vi "CRYGet Window Temp Reference.vi"(8 "sWindowName":string, 9 "sVIFullName":path, 10 "pVIRef_In":refnum<vi>, 11 "sAction":string) -> (0 "bResult":bool=TRUE, 1 "nWinType":i32, 2 "sTitleName Out":string, 3 "pVIRef_Out":refnum<vi>, 4 "sIcon_Out":string)   [LabVIEW 2013]
uses:
  <vilib>/Utility/miscctls.llb/LVPointTypeDef.ctl
  CRYWindow/SubVI/CRYMain Sub Window Global.vi
  Program/CRYRef nums global.vi
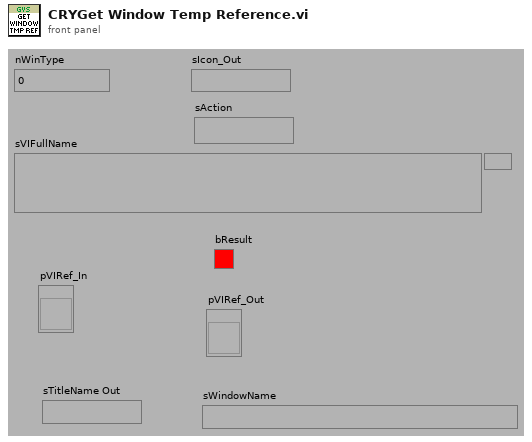
[diagram p1: front panel]
types:
  T1 = enum32{"Invalid", "Default", "Floating", "Floating/Auto-Hide", "Modal"}
  T2 = enum32{"Invalid", "Standard", "Closed", "Hidden", "Minimized", "Maximized"}
  T3 = typedef "LVPointTypeDef.ctl" = cluster{"Horizontal":i16, "Vertical":i16}
  T4 = cluster{"CLOSE_HIDE":i32, "CLOSE_CLOSE":i32, "DOCK_ENABLE":i32, "DOCK_DISABLE":i32, "FOCUS_SHOW":i32, "FOCUS_HIDE":i32}
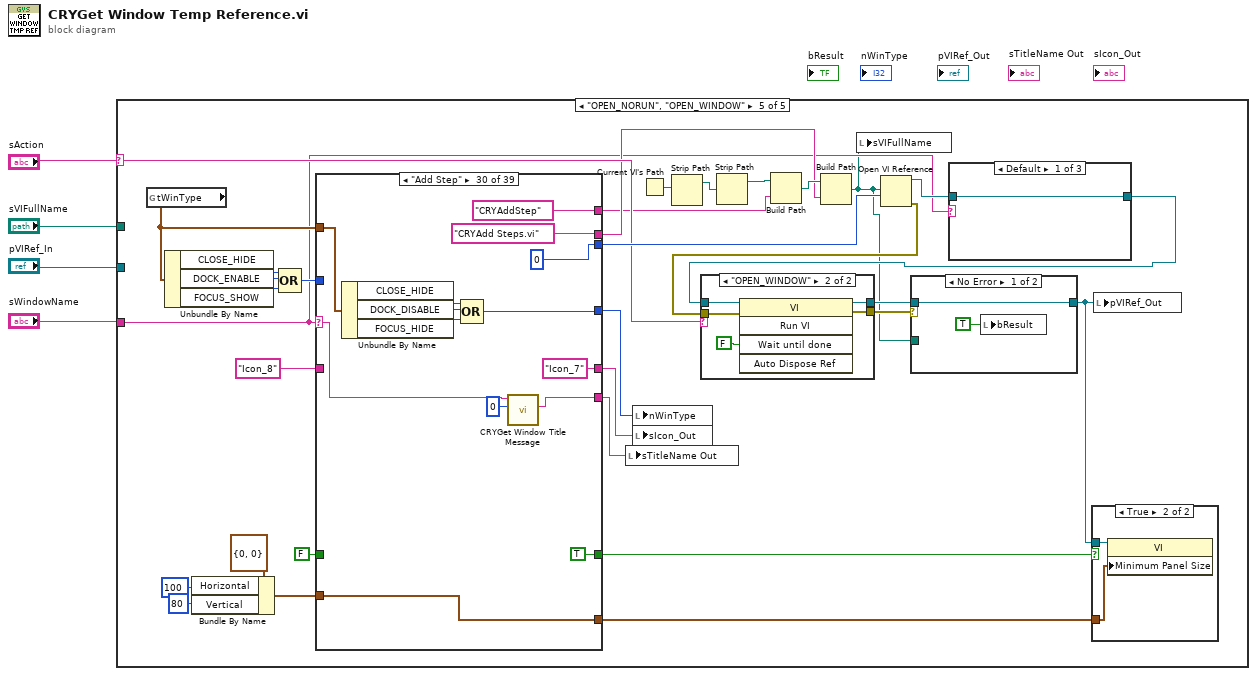
[diagram p0: block diagram]
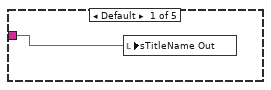
[diagram p2: hidden frame]
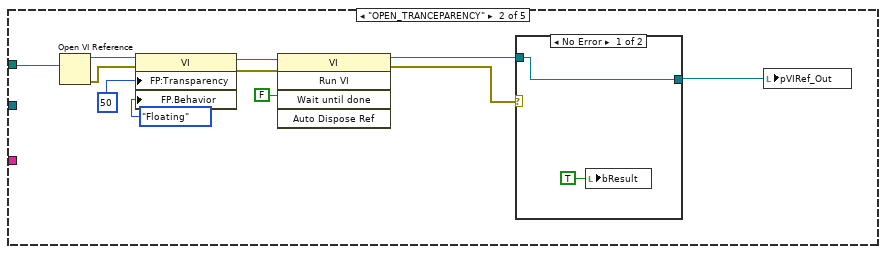
[diagram p3: hidden frame]
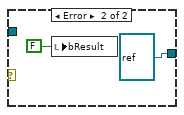
[diagram p4: hidden frame]
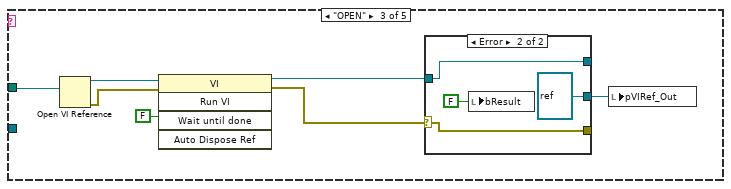
[diagram p5: hidden frame]
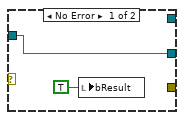
[diagram p6: hidden frame]
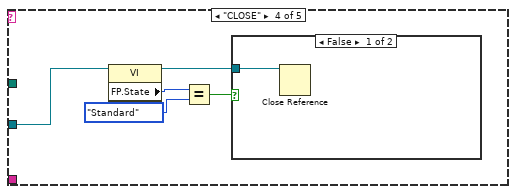
[diagram p7: hidden frame]
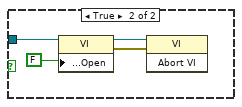
[diagram p8: hidden frame]
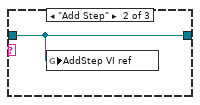
[diagram p9: hidden frame]
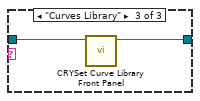
[diagram p10: hidden frame]
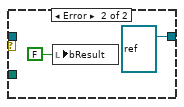
[diagram p13: hidden frame]
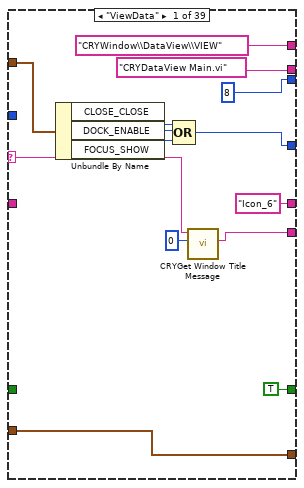
[diagram p14: hidden frame]
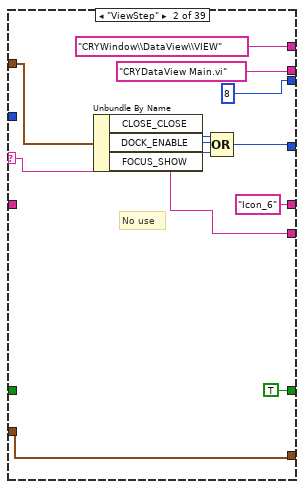
[diagram p15: hidden frame]
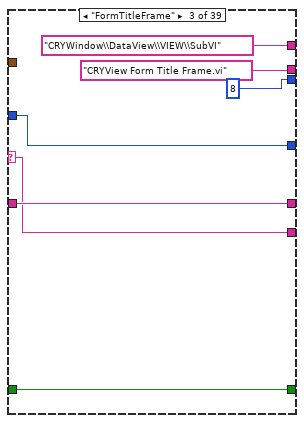
[diagram p16: hidden frame]
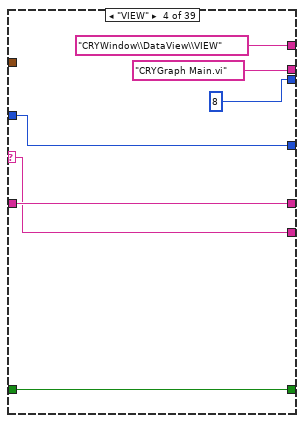
[diagram p17: hidden frame]
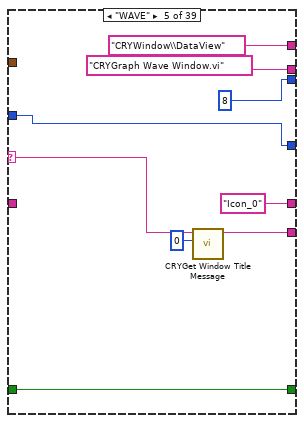
[diagram p18: hidden frame]
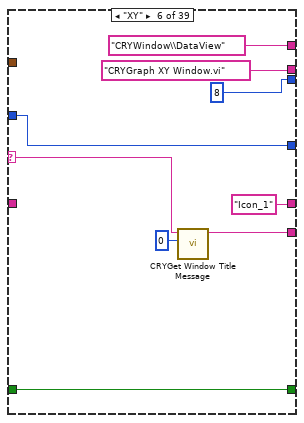
[diagram p19: hidden frame]
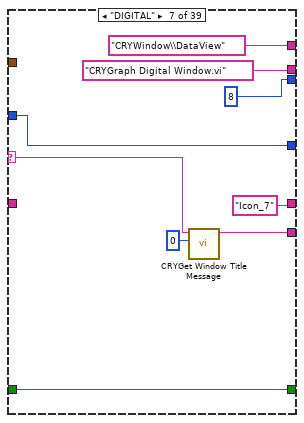
[diagram p20: hidden frame]
diagram:
  n1 = case shown="\"OPEN_NORUN\", \"OPEN_WINDOW\"" "sAction" {
    selector: "sAction" -> [_ _ _ _ w63]
    tunnel: "sVIFullName" -> [_ w7 w24 _ _]
    tunnel: "pVIRef_In" -> [_ _ _ w36 _]
    tunnel: "sWindowName" -> [w5 _ _ _ w48]
    frame Default {
      n2 = local write "sTitleName Out"(w5) -> ()
    }
    frame "OPEN_TRANCEPARENCY" {
      n3 = Open VI Reference(vi path=w7) -> (vi reference=w12:refnum<vi>, error out=w13:errorcluster)  [unwired: 1 in, 4 out]
      n4 = property class="VI"(reference=w12, error in=w13, "FP:Transparency"=u8 50 ("Front Panel Window:Transparency"), "FP.Behavior"=T1."Floating" ("Front Panel Window:Behavior")) -> (reference out=w15:refnum<vi>, error out=w16:errorcluster)
      n5 = invoke class="VI" method="Run VI"(reference=w15, error in=w16, "Wait until done"=FALSE ("Wait Until Done")) -> (reference out=w8:refnum<vi>, error out=w9:errorcluster)  [unwired: 2 in, 3 out]
      n6 = case shown="No Error" w9 {
        tunnel: w8 -> [w17 _]
        tunnel: [w17 refnum<vi> refnum ("VIRef")] -> w6
        frame No Error {
          n7 = local write "bResult"(TRUE ("bResult")) -> ()
        }
        frame Error {
          n8 = local write "bResult"(FALSE ("bResult")) -> ()
        }
      }
      n9 = local write "pVIRef_Out"(w6) -> ()
    }
    frame "OPEN" {
      n10 = Open VI Reference(vi path=w24) -> (vi reference=w23:refnum<vi>, error out=w22:errorcluster)  [unwired: 1 in, 4 out]
      n11 = invoke class="VI" method="Run VI"(reference=w23, error in=w22, "Wait until done"=FALSE ("Wait Until Done")) -> (reference out=w25:refnum<vi>, error out=w26:errorcluster)  [unwired: 2 in, 3 out]
      n12 = case shown="Error" w26 {
        selector: w26 -> [_ w30]
        tunnel: w25 -> [w28 w31]
        tunnel: [w28 refnum<vi> refnum ("VIRef_Out")] -> w21
        tunnel: [_ w31] -> _
        tunnel: [_ w30] -> _
        frame No Error {
          n13 = local write "bResult"(TRUE ("bResult")) -> ()
        }
        frame Error {
          n14 = local write "bResult"(FALSE ("bResult")) -> ()
        }
      }
      n15 = local write "pVIRef_Out"(w21) -> ()
    }
    frame "CLOSE" {
      n16 = property class="VI"(reference=w36) -> (reference out=w34:refnum<vi>, "FP.State"=w38:T2)  [unwired: 1 in, 1 out]
      n17 = Equal?(x=w38, y=T2."Standard" ("Front Panel Window:State")) -> (x = y?=w35:bool)
      n18 = case shown="False" w35 {
        tunnel: w34 -> [w39 w42]
        frame False {
          n19 = Close Reference(reference=w39) -> ()  [unwired: 1 in, 1 out]
        }
        frame True {
          n20 = property class="VI"(reference=w42, "Front Panel.Open"=FALSE ("Front Panel Window:Open")) -> (reference out=w41:refnum<vi>, error out=w40:errorcluster)  [unwired: 1 in]
          n21 = invoke class="VI" method="Abort VI"(reference=w41, error in=w40) -> ()  [unwired: 1 in, 3 out]
        }
      }
    }
    frame "OPEN_NORUN", "OPEN_WINDOW" {
      n22 = global read "CRYMain Sub Window Global.vi" "tWinType"() -> (w61:T4)
      n23 = Unbundle By Name(w61) -> ("CLOSE_HIDE"=w68:i32, "DOCK_ENABLE"=w69:i32, "FOCUS_SHOW"=w70:i32)
      n24 = Bundle By Name(cluster=T3 {"Horizontal"=0, "Vertical"=0} ("Front Panel Window:Minimum Size"), "Horizontal"=i16 100, "Vertical"=i16 80) -> (w52:T3)
      n25 = Compound Arithmetic op=OR(w68, w69, w70) -> (w67:i32)
      n26 = case shown="\"Add Step\"" w48 {
        selector: w48 -> [w97 w109 w120 w128 w135 w144 w153 w162 w171 w180 w189 w198 w207 w216 w226 w234 w246 w259 w269 w279 w286 w293 w300 w309 w317 w328 w339 w350 w361 w370 w382 w391 w403 w410 w417 w424 w431 w438 w445]
        tunnel: ["CRYWindow\\DataView\\VIEW" ("name") "CRYWindow\\DataView\\VIEW" ("name") "CRYWindow\\DataView\\VIEW\\SubVI" ("name") "CRYWindow\\DataView\\VIEW" ("name") "CRYWindow\\DataView" ("name") "CRYWindow\\DataView" ("name") "CRYWindow\\DataView" ("name") "CRYWindow\\DataView" ("name") "CRYWindow\\DataView" ("name") "CRYWindow\\DataView" ("name") "CRYWindow\\DataView" ("name") "CRYWindow\\DataView" ("name") "CRYWindow\\DataView" ("name") "CRYWindow\\DataView" ("name") "CRYStepSetup" ("name") "CRYStepSetup" ("name") "CRYDocument" ("name") "CRYDocument" ("name") "CRYCurveLibrary" ("name") "CRYCurveLibrary\\SubVI" ("name") "CRYCurveLibrary\\SubVI" ("name") "CRYCurveLibrary\\SubVI" ("name") "CRYCurveLibrary\\SubVI" ("name") "CRYProject" ("name") "CRYSystem\\Misc" ("name") "CRYSystem\\Misc" ("name") "CRYSystem\\Misc" ("name") "CRYSystem\\Misc" ("name") "CRYWindow\\SubVI" ("name") "CRYAddStep" ("name") "CRYOne\\" ("name") "CRYOne" ("name") "CRYWindow\\SubVI" ("name") "CRYWindow\\SubVI" ("name") "CRYWindow\\SubVI" ("name") "CRYWindow\\SubVI" ("name") "CRYWindow\\SubVI" ("name") "CRYSystem\\Misc" ("name") "CRYWindow\\SubVI" ("name")] -> w51
        tunnel: ["CRYDataView Main.vi" ("name") "CRYDataView Main.vi" ("name") "CRYView Form Title Frame.vi" ("name") "CRYGraph Main.vi" ("name") "CRYGraph Wave Window.vi" ("name") "CRYGraph XY Window.vi" ("name") "CRYGraph Digital Window.vi" ("name") "CRYGraph Octave Window.vi" ("name") "CRYGraph Polar Window.vi" ("name") "CRYGraph Text Window.vi" ("name") "CRYGraph Table Window.vi" ("name") "CRYGraph Picture Window.vi" ("name") "CRYGraph Result Window.vi" ("name") "CRYGraph Intensity Window.vi" ("name") "CRYStepSetup.vi" ("name") "CRYStep Setup Default Window.vi" ("name") "CRYReport Main.vi" ("name") "SubVI\\CRYReport Frame.vi" ("name") "CRYCurve Library.vi" ("name") "CRYProbe Curve.vi" ("name") "CRYProbe Value.vi" ("name") "CRYProbe Result.vi" ("name") "CRYProbe Waveform.vi" ("name") "CRYProject Editor.vi" ("name") "CRYSignal Generator.vi" ("name") "CRYMultimeter.vi" ("name") "CRYScope-FFT.vi" ("name") "CRYRTA.vi" ("name") "CRYAPI TAB MAIN.vi" ("name") "CRYAdd Steps.vi" ("name") "CRYOne Quick Lunch Menu.vi" ("name") "CRYSequence Generator.vi" ("name") "CRYAPI Splitter Vertical.vi" ("name") "CRYAPI Splitter Horizontal.vi" ("name") "CRYAPI Temp Empty.vi" ("name") "CRYAPI Temp Frame.vi" ("name") "CRYAPI MSG PRO.vi" ("name") "CRYOperator Message.vi" ("name") "CRYAPI Temp Default.vi" ("name")] -> w60
        tunnel: [w99 w110 w123 w131 w140 w149 w158 w166 w175 w184 w193 w202 w211 w220 w228 w238 w248 w263 w272 w282 w289 w295 w303 w313 w318 w329 w340 w351 w364 w374 w385 w395 w406 0 w420 w427 w434 w441 w448] -> w71
        tunnel: w67 -> [_ _ w123 w131 w140 w149 w158 w166 w175 w184 w193 w202 w211 w220 w228 w238 _ w263 w272 w282 w289 w295 w303 w313 _ _ _ _ w364 _ w385 _ w406 _ w420 w427 w434 w441 w448]
        tunnel: "Icon_8" ("sIcon_Out") -> [_ _ w122 w130 _ _ _ _ _ _ _ _ _ _ _ w237 _ _ _ w281 w287 w294 w301 _ _ _ _ _ w363 _ w383 _ w405 w412 w419 w426 w433 w440 w447]
        tunnel: ["Icon_6" ("sIcon_Out") "Icon_6" ("sIcon_Out") w122 w130 "Icon_0" ("sIcon_Out") "Icon_1" ("sIcon_Out") "Icon_7" ("sIcon_Out") "Icon_5" ("sIcon_Out") "Icon_2" ("sIcon_Out") "Icon_6" ("sIcon_Out") "Icon_3" ("sIcon_Out") "Icon_8" ("sIcon_Out") "Icon_4" ("sIcon_Out") "Icon_9" ("sIcon_Out") "Icon_3" ("sIcon_Out") w237 "Icon_4" ("sIcon_Out") "Icon_6" ("sIcon_Out") w264 w281 w287 w294 w301 "Icon_1" ("sIcon_Out") "Icon_8" ("sIcon_Out") "Icon_8" ("sIcon_Out") "Icon_8" ("sIcon_Out") "Icon_8" ("sIcon_Out") w363 "Icon_7" ("sIcon_Out") w383 "Icon_7" ("sIcon_Out") w405 w412 w419 w426 w433 w440 w447] -> w65
        tunnel: [8 ("options") 8 ("options") 8 ("options") 8 ("options") 8 ("options") 8 ("options") 8 ("options") 8 ("options") 8 ("options") 8 ("options") 8 ("options") 8 ("options") 8 ("options") 8 ("options") 8 ("options") 8 ("options") 8 ("options") 8 ("options") 0 ("options") 8 ("options") 8 ("options") 8 ("options") 8 ("options") 0 ("options") 8 ("options") 8 ("options") 8 ("options") 8 ("options") 8 ("options") 0 ("options") 0 ("options") 0 ("options") 8 ("options") 8 ("options") 8 ("options") 8 ("options") 8 ("options") 0 ("options") 8 ("options")] -> w64
        tunnel: w61 -> [w100 w111 _ _ _ _ _ _ _ _ _ _ _ _ _ _ w249 _ _ _ _ _ _ _ w319 w330 w341 w352 _ w375 _ w396 _ _ _ _ _ _ _]
        tunnel: [w96 w109 w120 w128 w133 w142 w151 w160 w169 w178 w187 w196 w205 w214 w225 w234 w245 w259 w268 w279 w286 w293 w300 w308 w317 w328 w339 w350 w361 w369 w382 w390 w403 w410 w417 w424 w431 w438 w445] -> w62
        tunnel: FALSE -> [_ _ w119 w127 w134 w143 w152 w161 w170 w179 w188 w197 w206 w215 _ w233 _ w257 _ w278 w285 w292 w299 _ w316 w327 w338 w349 w360 _ w381 _ w402 w409 w416 w423 w430 w437 w444]
        tunnel: [TRUE TRUE w119 w127 w134 w143 w152 w161 w170 w179 w188 w197 w206 w215 TRUE w233 TRUE w257 TRUE w278 w285 w292 w299 TRUE w316 w327 w338 w349 w360 TRUE w381 TRUE w402 w409 w416 w423 w430 w437 w444] -> w57
        tunnel: [w94 w107 _ _ _ _ _ _ _ _ _ _ _ _ w223 _ w241 _ w266 _ _ _ _ w306 _ _ _ _ _ w367 _ w388 _ _ _ _ _ _ _] -> w56
        tunnel: w52 -> [w94 w107 _ _ _ _ _ _ _ _ _ _ _ _ w223 _ _ _ w266 _ _ _ _ w306 _ _ _ _ _ w367 _ w388 _ _ _ _ _ _ _]
        frame "ViewData" {
          n27 = Unbundle By Name(w100) -> ("CLOSE_CLOSE"=w103:i32, "DOCK_ENABLE"=w102:i32, "FOCUS_SHOW"=w101:i32)
          n28 = Compound Arithmetic op=OR(w103, w102, w101) -> (w99:i32)
          n29 = call "CRYGet Window Title Message.vi"("No"=0 ("Error No"), "Kind"=w97) -> ("Unicode String"=w96:string)  [unwired: 4 in, 5 out]
        }
        frame "ViewStep" {
          # "No use"
          n30 = Unbundle By Name(w111) -> ("CLOSE_CLOSE"=w114:i32, "DOCK_ENABLE"=w113:i32, "FOCUS_SHOW"=w112:i32)
          n31 = Compound Arithmetic op=OR(w114, w113, w112) -> (w110:i32)
        }
        frame "FormTitleFrame" {
        }
        frame "VIEW" {
        }
        frame "WAVE" {
          n32 = call "CRYGet Window Title Message.vi"("No"=0 ("Error No"), "Kind"=w135) -> ("Multibyte String"=w133:string)  [unwired: 4 in, 5 out]
        }
        frame "XY" {
          n33 = call "CRYGet Window Title Message.vi"("No"=0 ("Error No"), "Kind"=w144) -> ("Multibyte String"=w142:string)  [unwired: 4 in, 5 out]
        }
        frame "DIGITAL" {
          n34 = call "CRYGet Window Title Message.vi"("No"=0 ("Error No"), "Kind"=w153) -> ("Multibyte String"=w151:string)  [unwired: 4 in, 5 out]
        }
        frame "OCTAVE" {
          n35 = call "CRYGet Window Title Message.vi"("No"=0 ("Error No"), "Kind"=w162) -> ("Multibyte String"=w160:string)  [unwired: 4 in, 5 out]
        }
        frame "POLAR" {
          n36 = call "CRYGet Window Title Message.vi"("No"=0 ("Error No"), "Kind"=w171) -> ("Multibyte String"=w169:string)  [unwired: 4 in, 5 out]
        }
        frame "TEXT" {
          n37 = call "CRYGet Window Title Message.vi"("No"=0 ("Error No"), "Kind"=w180) -> ("Multibyte String"=w178:string)  [unwired: 4 in, 5 out]
        }
        frame "TABLE" {
          n38 = call "CRYGet Window Title Message.vi"("No"=0 ("Error No"), "Kind"=w189) -> ("Multibyte String"=w187:string)  [unwired: 4 in, 5 out]
        }
        frame "PICTURE" {
          n39 = call "CRYGet Window Title Message.vi"("No"=0 ("Error No"), "Kind"=w198) -> ("Multibyte String"=w196:string)  [unwired: 4 in, 5 out]
        }
        frame "RESULT" {
          n40 = call "CRYGet Window Title Message.vi"("No"=0 ("Error No"), "Kind"=w207) -> ("Multibyte String"=w205:string)  [unwired: 4 in, 5 out]
        }
        frame "INTENSITY" {
          n41 = call "CRYGet Window Title Message.vi"("No"=0 ("Error No"), "Kind"=w216) -> ("Multibyte String"=w214:string)  [unwired: 4 in, 5 out]
        }
        frame "Step Setup" {
          n42 = call "CRYGet Window Title Message.vi"("No"=0 ("Error No"), "Kind"=w226) -> ("Unicode String"=w225:string)  [unwired: 4 in, 5 out]
        }
        frame "Step Setup Default" {
        }
        frame "Document" {
          n43 = Unbundle By Name(w249) -> ("CLOSE_CLOSE"=w252:i32, "DOCK_ENABLE"=w251:i32, "FOCUS_SHOW"=w250:i32)
          n44 = Bundle By Name(cluster=T3 {"Horizontal"=0, "Vertical"=0} ("Front Panel Window:Minimum Size"), "Horizontal"=i16 300, "Vertical"=i16 200) -> (w241:T3)
          n45 = Compound Arithmetic op=OR(w252, w251, w250) -> (w248:i32)
          n46 = call "CRYGet Window Title Message.vi"("No"=0 ("Error No"), "Kind"=w246) -> ("Unicode String"=w245:string)  [unwired: 4 in, 5 out]
        }
        frame "ReportFrame" {
        }
        frame "Curves Library" {
          n47 = disable-structure shown="Enabled" {
            disable-tunnel: [w275 0 ("No")] -> w265
            disable-tunnel: [w274 "Icon_2" ("sIcon_Out")] -> w264
            frame Disabled {
              n48 = call "CRYGet Title Name and Icon from Type.vi"() -> ("Icon Name"=w274:string, "Title No"=w275:i32)  [unwired: 10 in]
            }
            frame Enabled {
            }
          }
          n49 = call "CRYGet Window Title Message.vi"("No"=w265, "Kind"=w269) -> ("Unicode String"=w268:string)  [unwired: 4 in, 5 out]
        }
        frame "Probe Curve" {
        }
        frame "Probe Value" {
        }
        frame "Probe Result" {
        }
        frame "Probe Waveform" {
        }
        frame "Project" {
          n50 = call "CRYGet Window Title Message.vi"("No"=0 ("Error No"), "Kind"=w309) -> ("Unicode String"=w308:string)  [unwired: 4 in, 5 out]
        }
        frame "Signal Generator" {
          n51 = Unbundle By Name(w319) -> ("CLOSE_CLOSE"=w322:i32, "DOCK_DISABLE"=w321:i32, "FOCUS_SHOW"=w320:i32)
          n52 = Compound Arithmetic op=OR(w322, w321, w320) -> (w318:i32)
        }
        frame "Multimeter" {
          n53 = Unbundle By Name(w330) -> ("CLOSE_CLOSE"=w333:i32, "DOCK_DISABLE"=w332:i32, "FOCUS_SHOW"=w331:i32)
          n54 = Compound Arithmetic op=OR(w333, w332, w331) -> (w329:i32)
        }
        frame "Oscilloscope-FFT" {
          n55 = Unbundle By Name(w341) -> ("CLOSE_CLOSE"=w344:i32, "DOCK_DISABLE"=w343:i32, "FOCUS_SHOW"=w342:i32)
          n56 = Compound Arithmetic op=OR(w344, w343, w342) -> (w340:i32)
        }
        frame "RTA" {
          n57 = Unbundle By Name(w352) -> ("CLOSE_CLOSE"=w355:i32, "DOCK_DISABLE"=w354:i32, "FOCUS_SHOW"=w353:i32)
          n58 = Compound Arithmetic op=OR(w355, w354, w353) -> (w351:i32)
        }
        frame "TAB" {
        }
        frame "Add Step" {
          n59 = Unbundle By Name(w375) -> ("CLOSE_HIDE"=w378:i32, "DOCK_DISABLE"=w377:i32, "FOCUS_HIDE"=w376:i32)
          n60 = Compound Arithmetic op=OR(w378, w377, w376) -> (w374:i32)
          n61 = call "CRYGet Window Title Message.vi"("No"=0 ("Error No"), "Kind"=w370) -> ("Unicode String"=w369:string)  [unwired: 4 in, 5 out]
        }
        frame "Quick_Lunch_Menu" {
        }
        frame "Sequence Generator" {
          n62 = Unbundle By Name(w396) -> ("CLOSE_HIDE"=w399:i32, "DOCK_DISABLE"=w398:i32, "FOCUS_HIDE"=w397:i32)
          n63 = Compound Arithmetic op=OR(w399, w398, w397) -> (w395:i32)
          n64 = call "CRYGet Window Title Message.vi"("No"=0 ("Error No"), "Kind"=w391) -> ("Unicode String"=w390:string)  [unwired: 4 in, 5 out]
        }
        frame "MainVertSplitter" {
        }
        frame "MainHorizSplitter" {
        }
        frame "CenterEmpty" {
        }
        frame "BasicWindow" {
        }
        frame "MsgProcesser" {
        }
        frame "Operator Msg Proc" {
        }
        frame Default {
        }
      }
      n65 = local write "sTitleName Out"(w62) -> ()
      n66 = local write "nWinType"(w71) -> ()
      n67 = local write "sIcon_Out"(w65) -> ()
      n68 = Current VI's Path() -> (path=w47:path)
      n69 = Strip Path(path=w47) -> (stripped path=w46:path)  [unwired: 1 out]
      n70 = Strip Path(path=w46) -> (stripped path=w44:path)  [unwired: 1 out]
      n71 = Build Path(base path=w44, name or relative path=w51) -> (appended path=w75:path)
      n72 = Build Path(base path=w75, name or relative path=w60) -> (appended path=w45:path)
      n73 = local write "sVIFullName"(w45) -> ()
      n74 = Open VI Reference(vi path=w45, options=w64) -> (vi reference=w50:refnum<vi>, error out=w73:errorcluster)  [unwired: 1 in, 3 out]
      n75 = case shown="Default" w48 {
        tunnel: w50 -> [w76 w77 w79]
        tunnel: [w76 w77 w78] -> w49
        frame Default {
        }
        frame "Add Step" {
          n76 = global write "CRYRef nums global.vi" "AddStep VI ref"(w77) -> ()
        }
        frame "Curves Library" {
          n77 = call "CRYSet Curve Library Front Panel.vi"("Vi Ref In"=w79) -> ("Vi Ref Out"=w78:refnum<vi>)  [unwired: 10 in]
        }
      }
      n78 = case shown="\"OPEN_WINDOW\"" w63 {
        tunnel: [w82 w87] -> w74
        tunnel: w49 -> [w83 w86]
        tunnel: w73 -> [w82 w85]
        tunnel: [w83 w84] -> w72
        frame Default {
        }
        frame "OPEN_WINDOW" {
          n79 = invoke class="VI" method="Run VI"(reference=w86, error in=w85, "Wait until done"=FALSE ("Wait Until Done")) -> (reference out=w84:refnum<vi>, error out=w87:errorcluster)  [unwired: 2 in, 3 out]
        }
      }
      n80 = case shown="No Error" w74 {
        tunnel: [w89 refnum<vi> refnum ("VIRef_Out")] -> w59
        tunnel: w72 -> [w89 _]
        tunnel: w45 -> [_ _]
        frame No Error {
          n81 = local write "bResult"(TRUE ("bResult")) -> ()
        }
        frame Error {
          n82 = local write "bResult"(FALSE ("bResult")) -> ()
        }
      }
      n83 = case shown="True" w57 {
        tunnel: w59 -> [_ w81]
        tunnel: w56 -> [_ w80]
        frame False {
        }
        frame True {
          n84 = property class="VI"(reference=w81, "Minimum Panel Size"=w80) -> ()  [unwired: 1 in, 2 out]
        }
      }
      n85 = local write "pVIRef_Out"(w59) -> ()
    }
  }
